vi "Full experiment TIFF.vi"() -> ()   [LabVIEW 2018]
uses:
  <vilib>/userdefined/High Color/IMAQdx.ctl
  <vilib>/Platform/TimedLoop/XDataNode/nitl_modes.ctl
  <vilib>/Platform/TimedLoop/XDataNode/timing_clust.ctl
  <vilib>/Platform/TimedLoop/XDataNode/wakeup.ctl
  <vilib>/platform/TimedLoop/XDataNode/XDataNode.xnode
  <vilib>/vision/driver/NI_Vision_Acquisition_Software.lvlib
  <vilib>/Platform/TimedLoop/XDataNode/XDNodeRunTimeDep.lvlib
panel:
  out "x-y":dbl
  out "Number of Frames":u32
  in  "Choose folder to save experiment TIFFs":path
  in  "Rat ¹":i16
  out "Closing the experiment":bool
  out "Experiment":bool
  in  "Error massages":T1(tab)
  out "error message":string caption="Initialization error message"
  out "error message 2":string caption="Real time video-tracking error message"
  out "error message 3":string caption="Experiment video-tracking error message"
  out "error message 4":string caption="Closing the experiment error message"
  out "Real time video-tracking":bool
  out "Read LED Forward Bias in V":dbl
  out "Read LED Wavelength in nm":dbl
  out "Read Counts from machine":i32
  in  "Set Counts in amounts of counts\n(0 means INFINITY)":i32 format="%.0g"
  out "Read Duty Cycle from machine":i32
  in  "Set Duty Cycle in %":i32=5 format="%.0g"
  out "Read frequency from machine":i32
  in  "Set frequency in Hz":i32=20
  out "Read current from machine":dbl
  in  "Set current in ampere":sgl=1.0 caption="Set current in A"
  in  "Start experiment":bool
  in  "Stop experiment":bool
  out "Real Time image":T2(plugin-control)
  out "Initialization status":bool
  in  "Choose DC2100 Thorlabs":refnum<visa-resource-name>="ASRL0::INSTR" caption="resource name"
  in  "Choose camera":T3
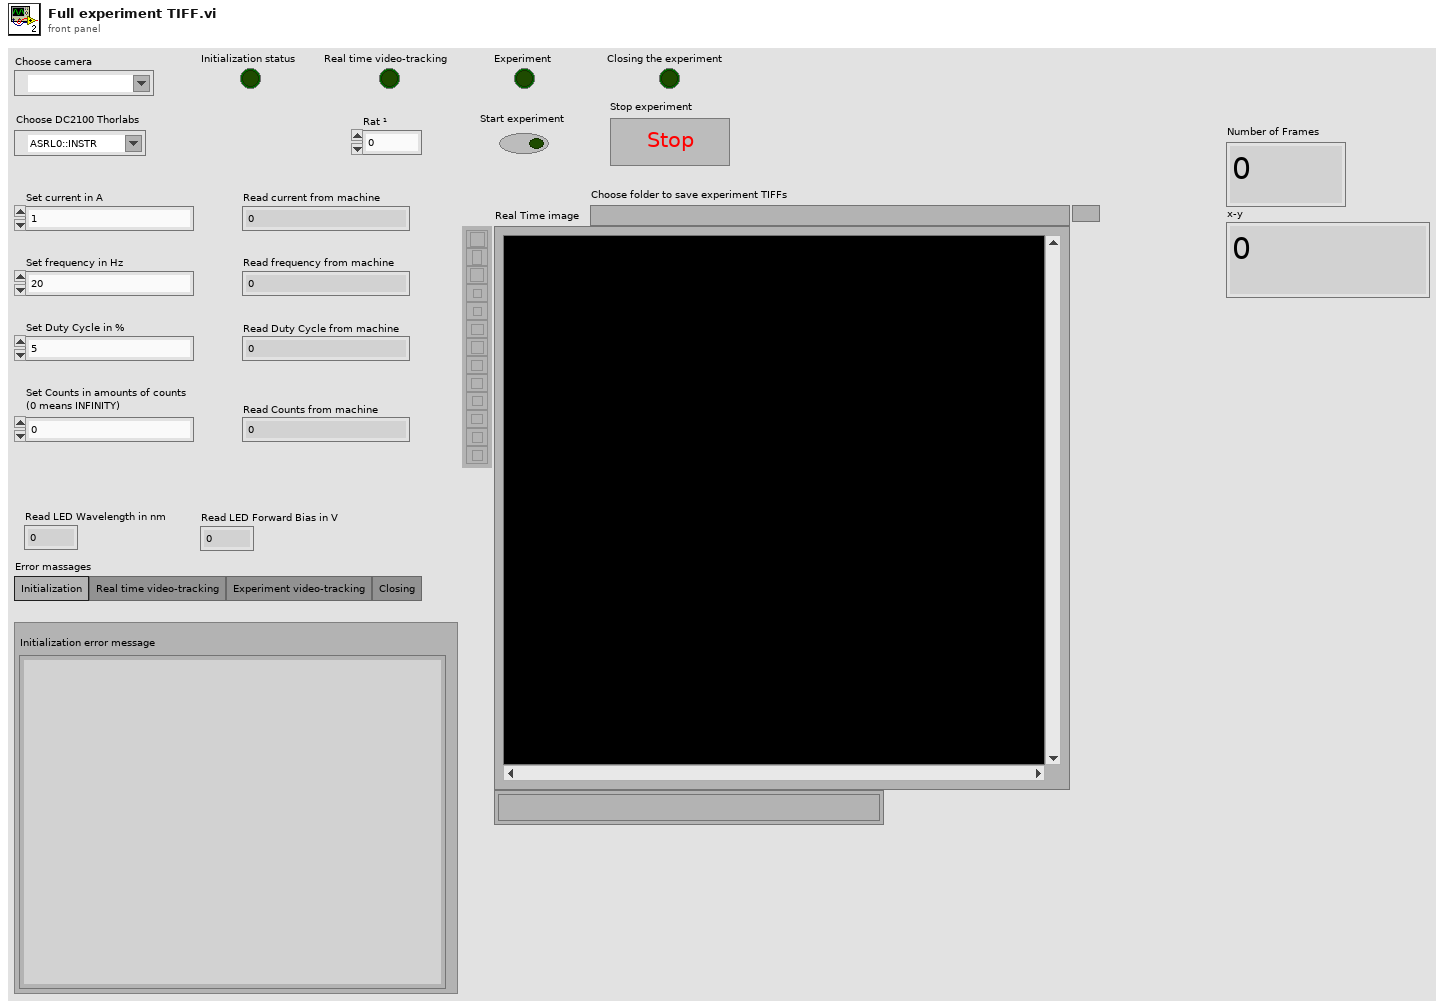
[diagram p1: front panel]
types:
  T1 = enum32{"Initialization", "Real time video-tracking", "Experiment video-tracking", "Closing"}
  T2 = typedef "IMAQ Image.ctl" = refnum<image>
  T3 = typedef "IMAQdx.ctl" = refnum<k21>
  T4 = typedef "XDNodeRunTimeDep.lvlib/nitl_modes.ctl" = enum32{"No Change", "Process missed periods, maintain original phase", "Discard missed periods, maintain original phase", "Process missed periods, ignore original phase", "Discard missed periods, ignore original phase"}
  T5 = typedef "XDNodeRunTimeDep.lvlib/timing_clust.ctl" = cluster{"Expected End [f-1]":u64, "Actual End [f-1]":u64, "Finished Late? [f-1]":bool, "Expected End [i-1]":u64, "Actual End [i-1]":u64, "Finished Late? [i-1]":bool, "Expected Start [i]":u64, "Actual Start [i]":u64, "Expected Start [f]":u64, "Actual Start [f]":u64, "Source Name":string, "Structure Name":string, "Period":i64, "Deadline":i64, "Offset":i64, "Start":i64, "Priority":i32, "Timeout":i32, "Mode":T4, "Wakeup Reason":T6, "Error":errorcluster, "Source Type":string, "Secondary Source Type":string, "Global End Time":u64, "Global Start Time":u64, "Frame Duration":u64, "Iteration Duration":u64, "Assigned CPU":i32, "I/O Scan Engine Mode":u32}
  T6 = typedef "XDNodeRunTimeDep.lvlib/wakeup.ctl" = enum32{"Normal", "Aborted", "Asynchronous wakeup", "Timing source error", "Timed loop error", "Timeout"}
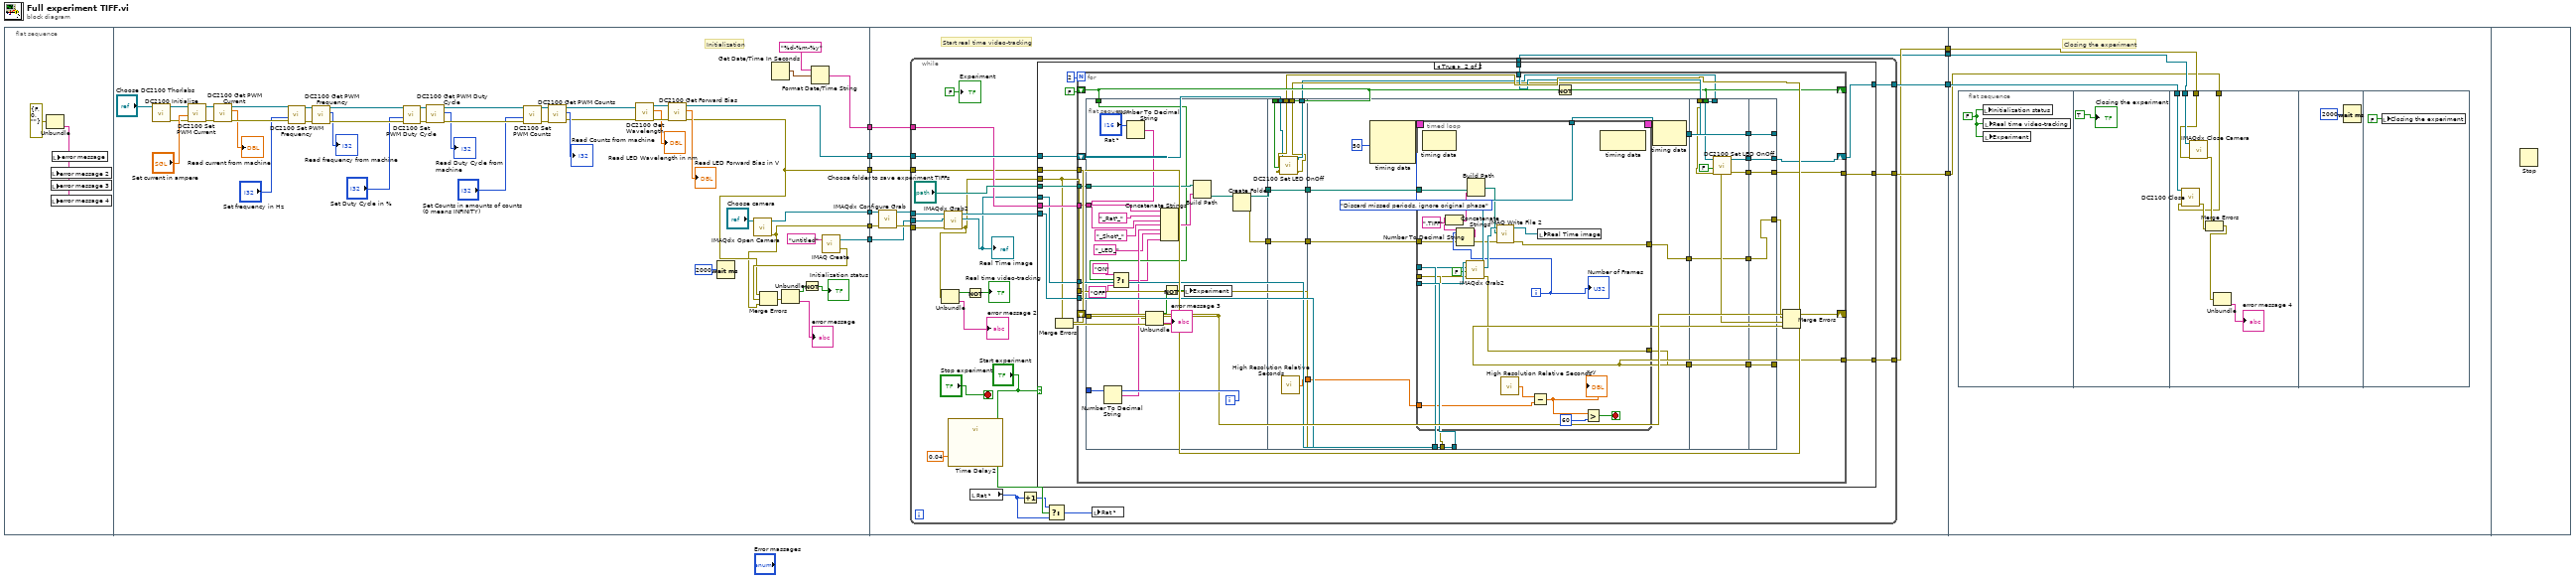
[diagram p0: block diagram]
diagram:
  n1 = flat-sequence {
    tunnel: [w56] -> w10
    tunnel: [w13] -> w9
    tunnel: [w23] -> w8
    tunnel: [w20] -> w7
    tunnel: [w15] -> w4
    tunnel: [w14] -> w3
    tunnel: w10 -> [w71]
    tunnel: w9 -> [w68]
    tunnel: w8 -> [w67]
    tunnel: w7 -> [w66]
    tunnel: [w65] -> w6
    tunnel: [w60] -> w5
    tunnel: w4 -> [w64]
    tunnel: w3 -> [w63]
    tunnel: [w61] -> w2
    tunnel: [w62] -> w1
    tunnel: w6 -> [w232]
    tunnel: w5 -> [w231]
    tunnel: w2 -> [w230]
    tunnel: w1 -> [w229]
    frame #0 {
      n2 = Unbundle(errorcluster {"status"=FALSE, "code"=0, "source"=""} ("error constant")) -> ("source"=w11:string)  [unwired: 2 out]
      n3 = local write "error message 2"(w11) -> ()
      n4 = local write "error message 3"(w11) -> ()
      n5 = local write "error message 4"(w11) -> ()
      n6 = local write "error message"(w11) -> ()
    }
    frame #1 {
      # "Initialization"
      n7 = call <instrlib>:"DC2100 Initialize.vi"("resource name"="Choose DC2100 Thorlabs") -> ("error out"=w27:errorcluster, "instrument handle out"=w28:refnum<visa-resource-name>)  [unwired: 9 in]
      n8 = call <instrlib>:"DC2100 Set PWM Current.vi"("error in (no error)"=w27, "Current (0.0)"="Set current in ampere", "instrument handle"=w28) -> ("error out"=w54:errorcluster, "instrument handle out"=w53:refnum<visa-resource-name>)  [unwired: 7 in]
      n9 = call <instrlib>:"DC2100 Get PWM Current.vi"("error in (no error)"=w54, "instrument handle"=w53) -> ("error out"=w44:errorcluster, "Current"=→"Read current from machine":dbl, "instrument handle out"=w45:refnum<visa-resource-name>)  [unwired: 7 in]
      n10 = call <instrlib>:"DC2100 Set PWM Frequency.vi"("error in (no error)"=w44, "Frequency (1)"="Set frequency in Hz", "instrument handle"=w45) -> ("error out"=w52:errorcluster, "instrument handle out"=w51:refnum<visa-resource-name>)  [unwired: 7 in]
      n11 = call <instrlib>:"DC2100 Get PWM Frequency.vi"("error in (no error)"=w52, "instrument handle"=w51) -> ("error out"=w42:errorcluster, "Frequency"=→"Read frequency from machine":i32, "instrument handle out"=w43:refnum<visa-resource-name>)  [unwired: 7 in]
      n12 = call <instrlib>:"DC2100 Set PWM Duty Cycle.vi"("error in (no error)"=w42, "Duty Cycle (1)"="Set Duty Cycle in %", "instrument handle"=w43) -> ("error out"=w50:errorcluster, "instrument handle out"=w49:refnum<visa-resource-name>)  [unwired: 7 in]
      n13 = call <instrlib>:"DC2100 Get PWM Duty Cycle.vi"("error in (no error)"=w50, "instrument handle"=w49) -> ("error out"=w40:errorcluster, "Duty Cycle"=→"Read Duty Cycle from machine":i32, "instrument handle out"=w41:refnum<visa-resource-name>)  [unwired: 7 in]
      n14 = call <instrlib>:"DC2100 Set PWM Counts.vi"("error in (no error)"=w40, "Counts (0)"="Set Counts in amounts of counts\n(0 means INFINITY)", "instrument handle"=w41) -> ("error out"=w48:errorcluster, "instrument handle out"=w47:refnum<visa-resource-name>)  [unwired: 7 in]
      n15 = call <instrlib>:"DC2100 Get PWM Counts.vi"("error in (no error)"=w48, "instrument handle"=w47) -> ("error out"=w24:errorcluster, "Counts"=→"Read Counts from machine":i32, "instrument handle out"=w25:refnum<visa-resource-name>)  [unwired: 7 in]
      n16 = call <instrlib>:"DC2100 Get Wavelength.vi"("error in (no error)"=w24, "instrument handle"=w25) -> ("error out"=w39:errorcluster, "Wavelength"=→"Read LED Wavelength in nm":dbl, "instrument handle out"=w38:refnum<visa-resource-name>)  [unwired: 7 in]
      n17 = call <instrlib>:"DC2100 Get Forward Bias.vi"("error in (no error)"=w39, "instrument handle"=w38) -> ("error out"=w15:errorcluster, "Forward Bias"=→"Read LED Forward Bias in V":dbl, "instrument handle out"=w23:refnum<visa-resource-name>)  [unwired: 7 in]
      n18 = Wait (ms)(milliseconds to wait=u32 2000) -> ()  [unwired: 1 out]
      n19 = call <vilib>:"IMAQdx Open Camera.vi"("Session In"="Choose camera") -> ("error out"=w14:errorcluster, "Session Out"=w56:T3)  [unwired: 9 in]
      n20 = Get Date/Time In Seconds() -> (seconds since 1Jan1904=w22:timestamp)
      n21 = Format Date/Time String(time format string (%c)="%d-%m-%y", seconds (now)=w22) -> (date/time string=w20:string)  [unwired: 1 in]
      n22 = call "IMAQ Create"("Image Name"="untitled") -> ("New Image"=w13:T2, "error out"=w16:errorcluster)  [unwired: 4 in]
      n23 = Merge Errors(w15, w16, w14) -> (w17:errorcluster)
      n24 = Unbundle(w17) -> ("status"=w18:bool, "source"=→"error message":string)  [unwired: 1 out]
      n25 = Not(x=w18) -> (.not. x?=→"Initialization status":bool)
    }
    frame #2 {
      # "Start real time video-tracking"
      n26 = call <vilib>:"IMAQdx Configure Grab.vi"("error in"=w63, "Session In"=w71) -> ("error out"=w70:errorcluster, "Session Out"=w69:T3)  [unwired: 8 in]
      n27 = while {
        tunnel: w70 -> [w95]
        tunnel: w69 -> [w94]
        tunnel: w68 -> [w93]
        tunnel: w67 -> [w89]
        tunnel: w66 -> [w87]
        tunnel: [w86] -> w65
        tunnel: w64 -> [w83]
        tunnel: [w82] -> w62
        tunnel: [w74] -> w61
        tunnel: [w73] -> w60
        stop <- "Stop experiment" stop-if-true
        n28 = call <vilib>:"IMAQdx Grab2.vi"("error in"=w95, "Image In"=w93, "Session In"=w94) -> ("error out"=w75:errorcluster, "Image Out"=w76:T2, "Session Out"=w77:T3)  [unwired: 5 in, 1 out]
        "Real Time image" <- w76
        n29 = Unbundle(w75) -> ("status"=w85:bool, "source"=→"error message 2":string)  [unwired: 1 out]
        n30 = call "Time Delay2"("Delay Time (s)"=0.04) -> ()  [unwired: 10 in, 1 out]
        n31 = Not(x=w85) -> (.not. x?=→"Real time video-tracking":bool)
        n32 = local read "Rat ¹"() -> (w78:i16)
        n33 = Increment(x=w78) -> (x+1=w80:i16)
        n34 = case shown="True" "Start experiment" {
          tunnel: w89 -> [w99 w109]
          tunnel: "Choose folder to save experiment TIFFs" -> [_ w111]
          tunnel: w87 -> [_ w110]
          tunnel: [w99 w108] -> w86
          tunnel: w83 -> [w98 w104]
          tunnel: [w98 w107] -> w82
          tunnel: w77 -> [w96 w102]
          tunnel: w76 -> [_ w101]
          tunnel: w75 -> [w97 w100]
          tunnel: [w97 w106] -> w74
          tunnel: [w96 w105] -> w73
          frame False {
          }
          frame True {
            n35 = Merge Errors(w104, w100) -> (w103:errorcluster)
            n36 = for {
              N: 2 -> [_]
              shift-right: [w130] -> _
              shift-left: FALSE -> [w140]
              tunnel: w111 -> [w145]
              tunnel: w110 -> [w144]
              shift-right: [w142] -> _
              shift-left: w103 -> [w141]
              shift-right: [w127] -> w108
              shift-left: w109 -> [w137]
              tunnel: w104 -> [w138]
              tunnel: [w128] -> w107
              tunnel: [w133] -> w106
              tunnel: [w132] -> w105
              tunnel: w102 -> [w136]
              tunnel: w101 -> [w135]
              tunnel: w100 -> [w134]
              i -> [w143]
              n37 = flat-sequence {
                tunnel: w145 -> [w166]
                tunnel: w144 -> [w165]
                tunnel: w143 -> [w159]
                tunnel: w140 -> [w156]
                tunnel: w141 -> [w151]
                tunnel: [w147] -> w116
                tunnel: [w146] -> w115
                tunnel: w140 -> [w174]
                tunnel: [w169] -> w139
                tunnel: w138 -> [w173]
                tunnel: w137 -> [w172]
                tunnel: [w171] -> w129
                tunnel: [w170] -> w131
                tunnel: [w168] -> w117
                tunnel: w116 -> [w168]
                tunnel: w115 -> [w167]
                tunnel: [w167] -> w114
                tunnel: w139 -> [w187]
                tunnel: w136 -> [w186]
                tunnel: w135 -> [w185]
                tunnel: w134 -> [w184]
                tunnel: [w183] -> w125
                tunnel: [w182] -> w124
                tunnel: [w181] -> w123
                tunnel: w117 -> [w176]
                tunnel: w114 -> [w175]
                tunnel: w125 -> [w217]
                tunnel: w124 -> [w223]
                tunnel: w123 -> [w222]
                tunnel: w131 -> [w221]
                tunnel: w130 -> [_]
                tunnel: w129 -> [w220]
                tunnel: [w223] -> w122
                tunnel: [w222] -> w121
                tunnel: [w219] -> w120
                tunnel: [w218] -> w119
                tunnel: [w217] -> w118
                tunnel: [w224] -> w126
                tunnel: [w225] -> w127
                tunnel: [w226] -> w128
                tunnel: [w227] -> w132
                tunnel: [w228] -> w133
                tunnel: w122 -> [w228]
                tunnel: w121 -> [w227]
                tunnel: w120 -> [w226]
                tunnel: w119 -> [w225]
                tunnel: w118 -> [w224]
                frame #0 {
                  n38 = Number To Decimal String(number=w159) -> (decimal integer string=w158:string)  [unwired: 1 in]
                  n39 = Select(t="ON", s=w156, f="OFF") -> (s? t:f=w153:string)
                  n40 = Number To Decimal String(number="Rat ¹") -> (decimal integer string=w162:string)  [unwired: 1 in]
                  n41 = Unbundle(w151) -> ("status"=w150:bool, "source"=→"error message 3":string)  [unwired: 1 out]
                  n42 = Concatenate Strings(w165, "_Rat¹_" ("string"), w162, "_Shot¹_" ("string"), w158, "_LED_" ("string"), w153) -> (w161:string)
                  n43 = Not(x=w150) -> (.not. x?=w149:bool)
                  n44 = local write "Experiment"(w149) -> ()
                  n45 = Build Path(base path=w166, name or relative path=w161) -> (appended path=w148:path)
                  n46 = Create Folder(path (use dialog)=w148) -> (created path=w147:path, error out=w146:errorcluster)  [unwired: 2 in, 1 out]
                }
                frame #1 {
                  n47 = call <instrlib>:"DC2100 Set LED OnOff.vi"("error in (no error)"=w173, "LED On/Off (Off)"=w174, "instrument handle"=w172) -> ("error out"=w170:errorcluster, "instrument handle out"=w171:refnum<visa-resource-name>)  [unwired: 7 in]
                  n48 = call <vilib>:"High Resolution Relative Seconds.vi"() -> ("relative seconds"=w169:dbl)
                }
                frame #2 {
                  n49 = node-c288(i64 50 ("Period"), nitl_modes."Discard missed periods, ignore original phase" ("Mode")) -> (w180:T5)  [unwired: 1 in]
                  n50 = timed-loop {
                    tunnel: [w196] -> w183
                    tunnel: w187 -> [w205]
                    tunnel: w186 -> [w203]
                    tunnel: w185 -> [w202]
                    tunnel: w184 -> [w201]
                    tunnel: [w200] -> w182
                    tunnel: [w199] -> w181
                    timing: w180 -> [_]
                    timing-out: [_] -> w179
                    tunnel: w176 -> [w194]
                    tunnel: w175 -> [w191]
                    i -> [w193]
                    stop <- w207 stop-if-true
                    n51 = node-c288() -> ()  [unwired: 1 in, 1 out]
                    n52 = Number To Decimal String(number=w193) -> (decimal integer string=w189:string)  [unwired: 1 in]
                    n53 = Concatenate Strings(w189, ".TIFF" ("string")) -> (w188:string)
                    n54 = call <vilib>:"IMAQdx Grab2.vi"("error in"=w201, "Wait for Next Buffer? (Yes)"=FALSE, "Image In"=w202, "Session In"=w203) -> ("error out"=w200:errorcluster, "Image Out"=w195:T2, "Session Out"=w199:T3)  [unwired: 4 in, 1 out]
                    n55 = Build Path(base path=w194, name or relative path=w188) -> (appended path=w192:path)
                    n56 = call-poly "IMAQ Write File 2"("error in (no error)"=w191, "File Path"=w192, "Image"=w195) -> ("error out"=w196:errorcluster, "Image Out (duplicate)"=w197:T2)  [unwired: 7 in]
                    n57 = call <vilib>:"High Resolution Relative Seconds.vi"() -> ("relative seconds"=w206:dbl)
                    n58 = Subtract(x=w206, y=w205) -> (x-y=w204:dbl)
                    "x-y" <- w204
                    n59 = local write "Real Time image"(w197) -> ()
                    n60 = Greater?(x=w204, y=60) -> (0:w207:bool)
                    n61 = node-c288() -> ()  [unwired: 1 in, 1 out]
                    "Number of Frames" <- w193
                  }
                  n62 = node-c288(w179) -> ()  [unwired: 1 out]
                }
                frame #3 {
                  n63 = call <instrlib>:"DC2100 Set LED OnOff.vi"("error in (no error)"=w221, "LED On/Off (Off)"=FALSE, "instrument handle"=w220) -> ("error out"=w219:errorcluster, "instrument handle out"=w218:refnum<visa-resource-name>)  [unwired: 7 in]
                }
                frame #4 {
                }
              }
              n64 = Not(x=w140) -> (.not. x?=w130:bool)
              n65 = Merge Errors(w141, w126, w128, w133) -> (w142:errorcluster)
            }
          }
        }
        n66 = Select(t=w80, s="Start experiment", f=w78) -> (s? t:f=w79:i16)
        n67 = local write "Rat ¹"(w79) -> ()
        "Experiment" <- FALSE ("Experiment")
      }
    }
    frame #3 {
      # "Closing the experiment"
      n68 = flat-sequence {
        tunnel: w232 -> [w242]
        tunnel: w231 -> [w241]
        tunnel: w230 -> [w236]
        tunnel: w229 -> [w235]
        frame #0 {
          w233 = FALSE
          n69 = local write "Initialization status"(w233) -> ()
          n70 = local write "Real time video-tracking"(w233) -> ()
          n71 = local write "Experiment"(w233) -> ()
        }
        frame #1 {
          "Closing the experiment" <- TRUE
        }
        frame #2 {
          n72 = call <instrlib>:"DC2100 Close.vi"("error in (no error)"=w235, "instrument handle"=w242) -> ("error out"=w239:errorcluster)  [unwired: 9 in]
          n73 = call <vilib>:"IMAQdx Close Camera.vi"("error in"=w236, "Session In"=w241) -> ("error out"=w240:errorcluster)  [unwired: 9 in]
          n74 = Merge Errors(w240, w239) -> (w238:errorcluster)
          n75 = Unbundle(w238) -> ("source"=→"error message 4":string)  [unwired: 2 out]
        }
        frame #3 {
          n76 = Wait (ms)(milliseconds to wait=u32 2000) -> ()  [unwired: 1 out]
        }
        frame #4 {
          n77 = local write "Closing the experiment"(FALSE) -> ()
        }
      }
    }
    frame #4 {
      n78 = Stop() -> ()  [unwired: 1 in]
    }
  }
